vi "E816_Configuration_Setup No Password.vi"(0 "System no.":i32=1 min=1 step=1, 1 "Interface":u16(ring) items=["RS232", "USB"], 2 "Axes to move":string[](array[string]), 3 "All axes?":bool=TRUE, 4 "Change servo \nstatus to ON?":bool=TRUE, 5 "error in":errorcluster, 7 "Timeout":i32=5000, 8 "RS232 settings":cluster{"Portnumber":i32, "Baudrate":u16}={"Portnumber"=0, "Baudrate"=4} {"Portnumber" items=["COM1", "COM2", "COM3", "COM4", "COM5", "COM6", "COM7", "COM8", "COM9", "COM10", "COM11", "COM12", "COM13", "COM14", "COM15", "COM16", "COM17", "COM18", "COM19", "COM20", "COM21", "COM22", "COM23", "COM24", "COM25", "COM26", "COM27", "COM28", "COM29", "COM30"]; "Baudrate" items=["9600", "14400", "19200", "38400", "57600", "115200"]}, 9 "USB settings":cluster{"S/N":string, "USB Search?":bool}={"S/N"="", "USB Search?"=TRUE}, 13 "Stop refnum":refnum<vi>) -> (14 "Identification":string, 15 "SN out":string, 16 "Conn. Axes":string[](array[string]), 17 "Position":dbl[](array[numeric]) format="%.6f", 19 "error out":errorcluster)   [LabVIEW 2020]
doc: "This VI performs a fully automatic initialization of the selected system (global settings and servo status) in the LabVIEW environment. Use the Help?Show Context Help menu sequence in the LabVIEW environment to display the Context Help window with the VI and control/indicator descriptions.\n\nAfter the successful running of this VI, all command VIs are ready to use. Specify the correct parameters first: \n¢ System No.: 1 in a one-system-only configuration\n¢ Timeout value (in milliseconds)\n¢ Interface (RS232 or USB)\n¢ For Interface = RS232: RS-232 settings: Choose the port number the E-816 is connected to and an appropriate baud rate. \n¢ For Interface = USB: appropriate Serial Number of the controller to connect to or if you want to search for the controller.\n¢ Whether the servo status of all axes is to change to TRUE. If FALSE is selected here, the servo status will not be changed.\n\nThen start the VI.\n\"E816_Configuration_Setup.vi\" performs the following initialization tasks:\n1. Initializes all global variables.\n2. Runs \"PI Open Interface of one system.vi\" to open a connection to the controller. \n3. Runs \"*IDN?.vi\" to query for the controller identification string. \n4. Defines the selected system to be \"E-816\"\n5. Runs \"Define connected axes.vi\" with Read from controller = TRUE and Invert Order? = FALSE. \n6. Runs \"SVO.vi\" to switch servo ON for all connected axes if Change servo status to ON is TRUE.\n7. Runs \"SVO?.vi\" to query for the servo status of all connected axes.\n8. Runs \"POS?.vi\" to query for the position of all axes.\n9. Runs \"ERR?.vi\" to query the master controller for its error status.\n10. Runs \"GCSTranslateError.vi\" to append the error message which corresponds with a GCS error number returned by \"ERR?.vi\" to Source from Error out.\n\nUse this VI as the initialization VI for the E-816 in your application.\nWhen using as a sub-VI, connect Stop refnum terminal to stop VI from caller.\n\nAs the initialization is a complex procedure which uses a large number of sub-VIs, E816_Configuration_Setup.vi is password-protected, meaning that you cannot see or modify the diagram. In this way, the full initialization is packed into one single and fully tested procedure which you simply insert into your own application program. For security reasons as well as your convenience, we recommend that you not modify this VI."
uses:
  Low Level/Communication.llb/Available DLLs.ctl
  Low Level/Communication.llb/Available interfaces.ctl
  Low Level/Communication.llb/Available DLL interfaces.ctl
  Low Level/General command.llb/Controller names.ctl
  Low Level/Communication.llb/Global1.vi
panel:
  out "Servo status?":bool[](array[boolean])
  in  "Tab Control":enum32{"Interface settings", "Move settings"}(tab)
  in  "Frame":T1(ring)=enum."Open interface"
  in  "Finished":bool
  in  "stop":bool
  # "E-816 configuration setup program V6.0.2"
  # "This VI performs a full automatic initialization (global settings and servo status) for the\nselected system in the LabVIEW environment. After the successful run of this VI all \ncommand VIs are ready to use. Selectthe following settings first: interface settings and Move settings. See control/\nindicator information for details. Then start the VI. When using as a sub-VI, connect Stop refnum terminal to stop VI \nfrom caller.  See also VI information for details."
  # "Are all axes\nconnected\nand can be \nmoved?"
  # "If not:"
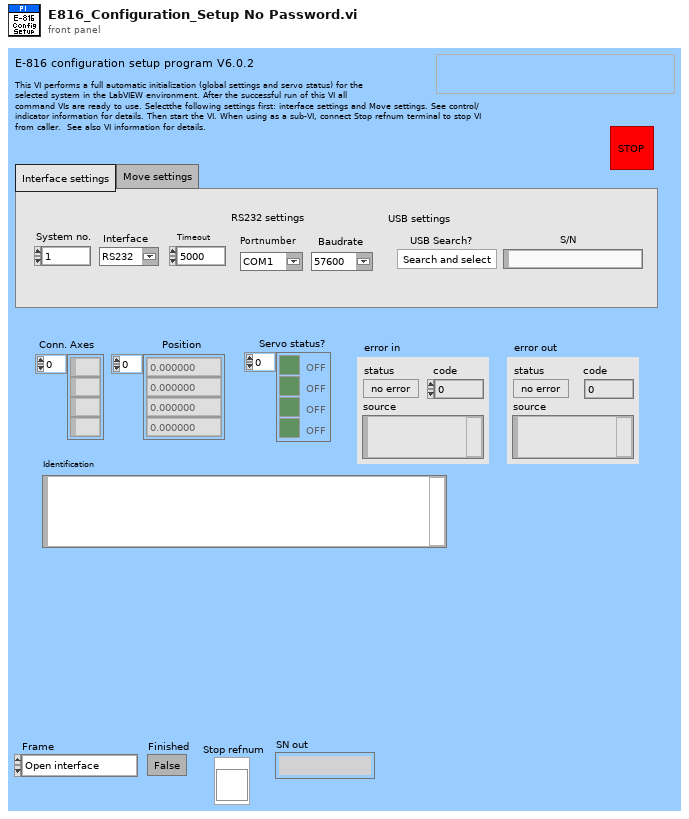
[diagram p1: front panel]
types:
  T1 = enum16{"Do nothing", "Initialize indicators", "Open interface", "Read IDs", "Set RON", "Reference", "Goto limit switch", "Move to middle", "Define home", "Translate error"}
  T2 = enum16{"DCO", "DCO?", "MOV", "MOV?", "MVR", "ONT?", "OVF?", "POS?", "RST", "SVA", "SVA?", "SVO", "SVO?", "SVR", "VOL?"}
  T3 = typedef "Available DLLs.ctl" = u16
  T4 = cluster{"input XON/XOFF":bool, "input HW Handshake":bool, "input alt HW HShk":bool, "output XON/XOFF":bool, "output HW Handshake":bool, "output alt HW HShk":bool, "XOFF byte ":u8, "XON byte":u8, "parity error byte":u16}[]
  T5 = typedef "Available DLL interfaces.ctl" = u16
  T6 = cluster{"input XON/XOFF":bool, "input HW Handshake":bool, "input alt HW HShk":bool, "output XON/XOFF":bool, "output HW Handshake":bool, "output alt HW HShk":bool, "XOFF byte ":u8, "XON byte":u8, "parity error byte":u16}
  T7 = typedef "Available interfaces.ctl" = u16
  T8 = cluster{"DLL for Device":T3, "DLL Interface":T5, "Parameter":string}[]
  T9 = cluster{"RS232 Portnumber":i32, "Timeout":i32, "RS232 Baud rate":u32, "Interface":T7, "GPIB Bus":i32, "GPIB Address":i32, "GPIB Mode":i32}[]
  T10 = cluster{"DLL for Device":T3, "DLL Interface":T5, "Parameter":string}
  T11 = cluster{"RS232 Portnumber":i32, "Timeout":i32, "RS232 Baud rate":u32, "Interface":T7, "GPIB Bus":i32, "GPIB Address":i32, "GPIB Mode":i32}
  T12 = typedef "Controller names.ctl" = enum16{"None", "Analog", "C-702", "C-843", "C-843.PM", "C-844", "C-848", "C-865", "C-866", "C-867", "C-880", "E-516", "E-517", "E-709", "E-710", "E-712", "E-725", "E-753", "E-755", "E-761", "E-816", "E-861", "F-206", "M-840", "M-850", "M-8X0", "Mercury", "Mercury_GCS"}
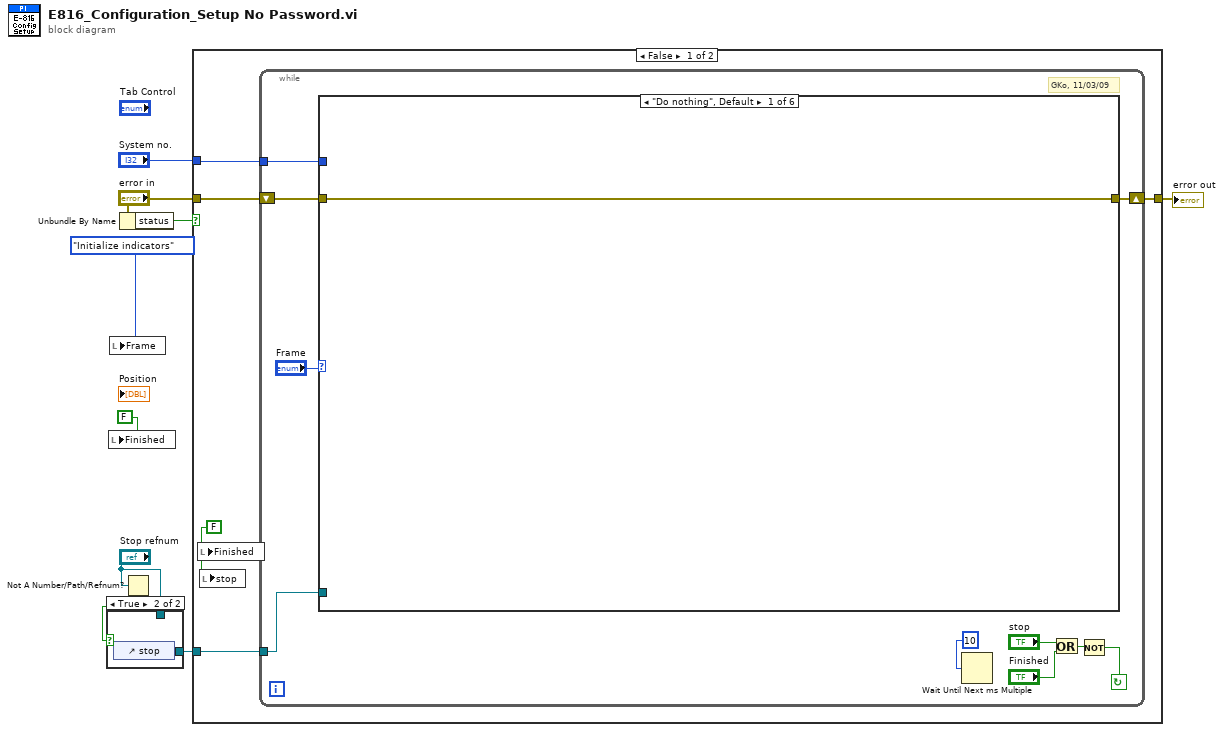
[diagram p0: block diagram]
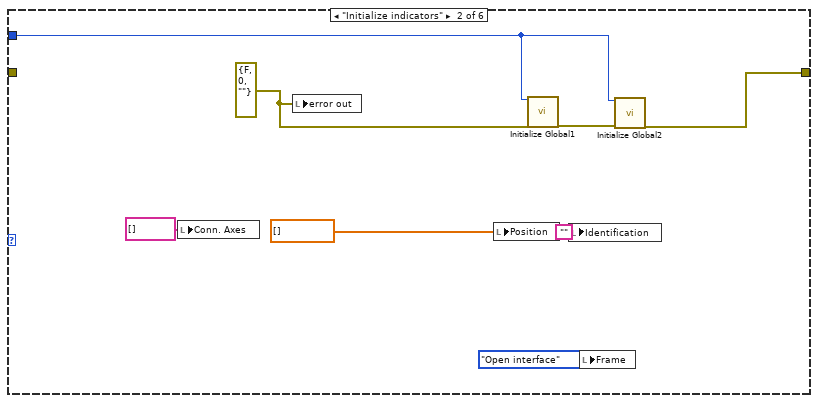
[diagram p3: hidden frame]
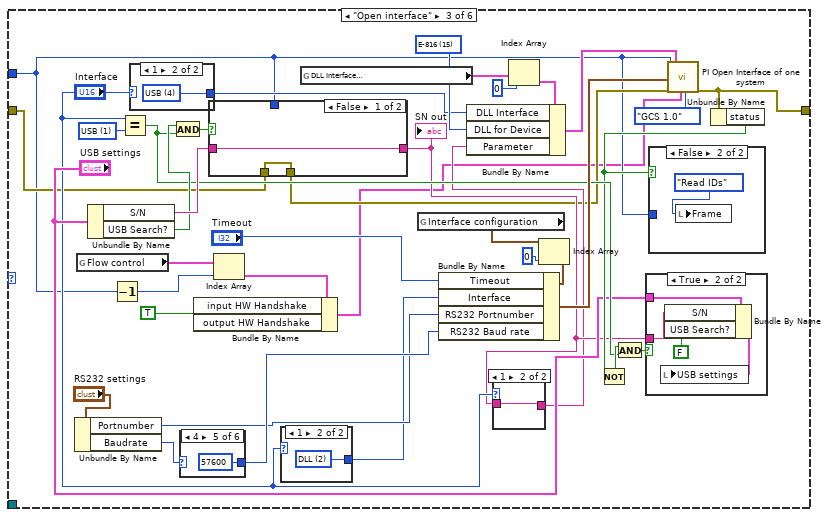
[diagram p4: hidden frame]
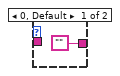
[diagram p5: hidden frame]
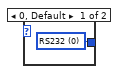
[diagram p6: hidden frame]
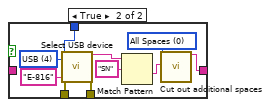
[diagram p8: hidden frame]
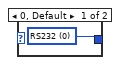
[diagram p9: hidden frame]
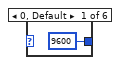
[diagram p10: hidden frame]
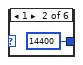
[diagram p11: hidden frame]
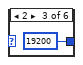
[diagram p12: hidden frame]
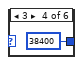
[diagram p13: hidden frame]
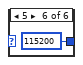
[diagram p14: hidden frame]
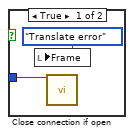
[diagram p15: hidden frame]
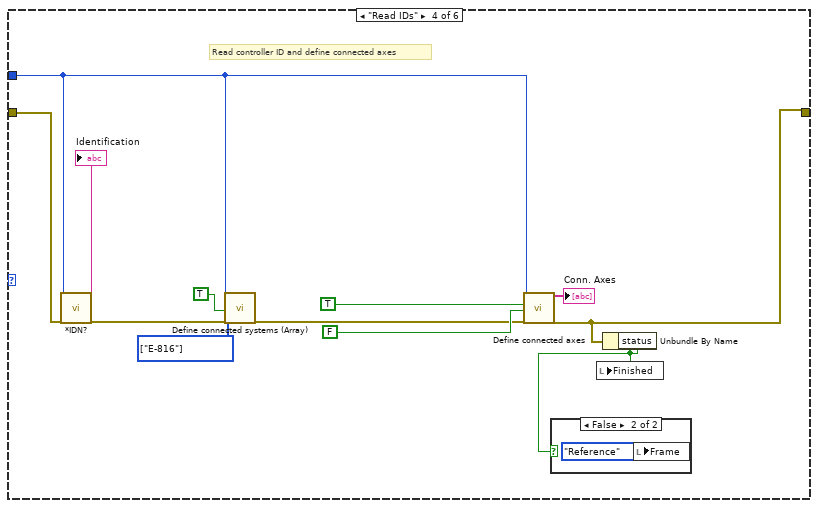
[diagram p16: hidden frame]
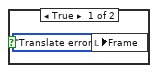
[diagram p17: hidden frame]
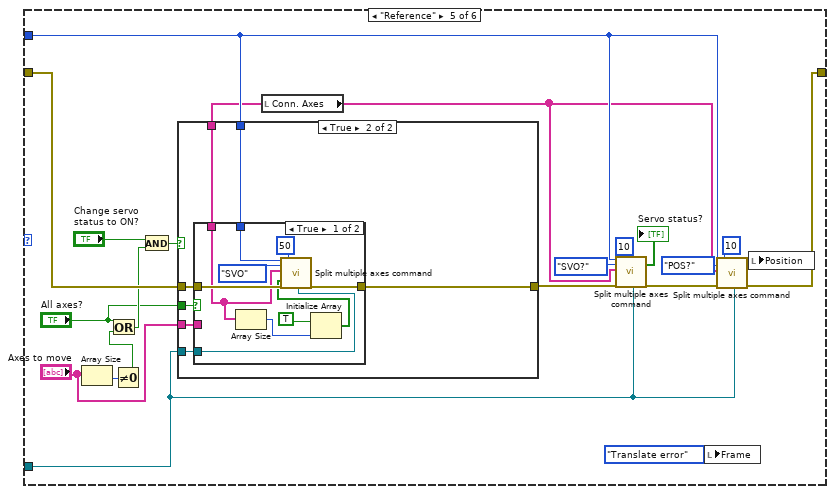
[diagram p18: hidden frame]
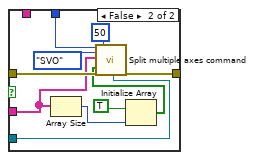
[diagram p20: hidden frame]
diagram:
  n1 = local write "Finished"(FALSE ("Finished")) -> ()
  n2 = local write "Frame"(T1."Initialize indicators" ("Frame")) -> ()
  n3 = Unbundle By Name("error in") -> ("status"=w8:bool)
  n4 = Not A Number/Path/Refnum?(number/path/refnum="Stop refnum") -> (NaN/Path/Refnum?=w4:bool)
  n5 = case shown="True" w4 {
    tunnel: [w10 w11] -> w2
    tunnel: "Stop refnum" -> [w10 _]
    frame False {
    }
    frame True {
      n6 = control-ref of="stop"() -> (w11:refnum<vi>)
    }
  }
  n7 = case shown="False" w8 {
    tunnel: [w15 w174] -> w6
    tunnel: "error in" -> [w16 w174]
    tunnel: "System no." -> [w14 _]
    tunnel: w2 -> [w12 _]
    frame False {
      w13 = FALSE ("Finished")
      n8 = local write "Finished"(w13) -> ()
      n9 = local write "stop"(w13) -> ()
      n10 = while {
        tunnel: w12 -> [w17]
        shift-left: w16 -> [w20]
        shift-right: [w19] -> w15
        tunnel: w14 -> [w18]
        stop <- w22 continue-if-true
        # "GKo, 11/03/09"
        n11 = case shown="\"Do nothing\", Default" "Frame" {
          tunnel: w18 -> [_ w29 w38 w107 w131 w169]
          tunnel: w20 -> [w27 _ w44 w110 w138 w172]
          tunnel: [w27 w30 w47 w106 w136 w170] -> w19
          tunnel: w17 -> [_ _ _ _ w124 _]
          frame "Do nothing", Default {
          }
          frame "Initialize indicators" {
            w31 = errorcluster {"status"=FALSE, "code"=0, "source"=""} ("error out")
            n12 = local write "Conn. Axes"(string[] [] ("Conn. Axes")) -> ()
            n13 = local write "error out"(w31) -> ()
            n14 = local write "Position"(dbl[] [] ("Position")) -> ()
            n15 = call "Initialize Global1.vi"("System no."=w29, "error in"=w31) -> ("error out"=w28:errorcluster)  [unwired: 17 in]
            n16 = local write "Identification"("" ("Identification")) -> ()
            n17 = local write "Frame"(T1."Open interface" ("Frame")) -> ()
            n18 = call "Initialize Global2.vi"("System no."=w29, "error in"=w28) -> ("error out"=w30:errorcluster)  [unwired: 17 in]
          }
          frame "Open interface" {
            w36 = u16 1 items=["RS232", "USB"] ("Interface")
            w64 = T3 15 items=["C-843", "C-844", "E-710", "C-843.PM", "C-865", "E-761", "Mercury", "E-755", "E-753", "C-866", "E-712", "E-725", "E-861", "C-867", "E-517", "E-816", "E-709", "PI_GCS2_DLL"] ("DLL for Device")
            w41 = TRUE ("Bundle Element")
            n19 = Unbundle By Name("RS232 settings") -> ("Portnumber"=w54:i32, "Baudrate"=w65:u16)
            n20 = global read "Global1.vi" "Flow control"() -> (w40:T4)
            n21 = Unbundle By Name("USB settings") -> ("S/N"=w63:string, "USB Search?"=w61:bool)
            n22 = Decrement(x=w38) -> (x-1=w39:i32)
            n23 = Equal?(x="Interface", y=w36) -> (x = y?=w57:bool)
            n24 = case shown="1" "Interface" {
              tunnel: [w94 w95] -> w56
              frame 0, Default {
                w94 = T5 0 items=["RS232", "GPIB", "Board", "TCP-IP", "USB", "RS232_DC"] ("DLL Interface")
              }
              frame 1 {
                w95 = T5 4 items=["RS232", "GPIB", "Board", "TCP-IP", "USB", "RS232_DC"] ("DLL Interface")
              }
            }
            n25 = And(x=w61, y=w57) -> (x .and. y?=w60:bool)
            n26 = case shown="4" w65 {
              tunnel: [9600 14400 19200 38400 57600 115200] -> w55
              frame 0, Default {
              }
              frame 1 {
              }
              frame 2 {
              }
              frame 3 {
              }
              frame 4 {
              }
              frame 5 {
              }
            }
            n27 = case shown="False" w60 {
              tunnel: [w83 w86] -> w49
              tunnel: w63 -> [w83 _]
              tunnel: w38 -> [_ w93]
              tunnel: w44 -> [w82 w90]
              tunnel: [w82 w89] -> w43
              frame False {
              }
              frame True {
                w87 = u16 0 items=["All Spaces", "Only if 1st char.", "Only if last char.", "Only if near \"=\"", "Only if 1st or last char.", "Only multiple", "Really all"] ("Mode")
                w92 = T5 4 items=["RS232", "GPIB", "Board", "TCP-IP", "USB", "RS232_DC"] ("DLL Interface")
                n28 = call "Select USB device.vi"("System no."=w93, "DLL Interface"=w92, "Controller name"="E-816", "error in"=w90) -> ("Selected USB controller"=w85:string, "error out"=w89:errorcluster)  [unwired: 13 in, 1 out]
                n29 = Match Pattern(string=w85, regular expression="SN") -> (after substring=w88:string)  [unwired: 4 out]
                n30 = call "Cut out additional spaces.vi"("String"=w88, "Mode"=w87) -> ("String out"=w86:string)  [unwired: 17 out]
              }
            }
            "SN out" <- w49
            n31 = Index Array(array=w40, index=w39) -> (element=w42:T6)
            n32 = Bundle By Name(cluster=w42, "input HW Handshake"=w41, "output HW Handshake"=w41) -> (w37:T6)
            n33 = case shown="1" "Interface" {
              tunnel: [w76 w77] -> w52
              frame 0, Default {
                w76 = T7 0 items=["RS232", "GPIB", "DLL", "TCP-IP", "USB", "Analog"] ("Interface")
              }
              frame 1 {
                w77 = T7 2 items=["RS232", "GPIB", "DLL", "TCP-IP", "USB", "Analog"] ("Interface")
              }
            }
            n34 = global read "Global1.vi" "DLL Interface\nConfiguration"() -> (w71:T8)
            n35 = global read "Global1.vi" "Interface configuration"() -> (w68:T9)
            n36 = case shown="1" "Interface" {
              tunnel: w49 -> [_ w75]
              tunnel: ["" w75] -> w48
              frame 0, Default {
              }
              frame 1 {
              }
            }
            n37 = Index Array(array=w71, index=0 ("Index")) -> (element=w72:T10)
            n38 = Bundle By Name(cluster=w72, "DLL Interface"=w56, "DLL for Device"=w64, "Parameter"=w48) -> (w67:T10)
            n39 = Index Array(array=w68, index=0 ("Index")) -> (element=w73:T11)
            n40 = Bundle By Name(cluster=w73, "Timeout"="Timeout", "Interface"=w52, "RS232 Portnumber"=w54, "RS232 Baud rate"=w55) -> (w66:T11)
            n41 = call "PI Open Interface of one system.vi"("System number"=w38, "Interface configuration"=w66, "error in"=w43, "DLL Interface\nConfiguration"=w67, "Flow control"=w37, "Syntax"=enum16{"GCS 1.0", "GCS 2.0"}."GCS 1.0") -> ("error out"=w47:errorcluster)  [unwired: 6 in, 7 out]
            n42 = Unbundle By Name(w47) -> ("status"=w53:bool)
            n43 = Not(x=w53) -> (.not. x?=w59:bool)
            n44 = And(x=w59, y=w57) -> (x .and. y?=w58:bool)
            n45 = case shown="True" w58 {
              tunnel: "USB settings" -> [_ w81]
              tunnel: w49 -> [_ w79]
              frame False {
              }
              frame True {
                n46 = Bundle By Name(cluster=w81, "S/N"=w79, "USB Search?"=FALSE) -> (w78:cluster{"S/N":string, "USB Search?":bool})
                n47 = local write "USB settings"(w78) -> ()
              }
            }
            n48 = case shown="False" w53 {
              tunnel: w38 -> [w103 _]
              frame True {
                n49 = local write "Frame"(T1."Translate error" ("Frame")) -> ()
                n50 = call "Close connection if open.vi"("System no."=w103) -> ()  [unwired: 17 in, 2 out]
              }
              frame False {
                n51 = local write "Frame"(T1."Read IDs" ("Frame")) -> ()
              }
            }
          }
          frame "Read IDs" {
            w105 = T12[] [enum."E-816"] items=["None", "Analog", "C-702", "C-843", "C-843.PM", "C-844", "C-848", "C-865", "C-866", "C-867", "C-880", "E-516", "E-517", "E-709", "E-710", "E-712", "E-725", "E-753", "E-755", "E-761", "E-816", "E-861", "F-206", "M-840", "M-850", "M-8X0", "Mercury", "Mercury_GCS"] ("Controller names")
            # "Read controller ID and define connected axes"
            n52 = call "*IDN?.vi"("System no."=w107, "error in"=w110) -> ("Identification"=→"Identification":string, "error out"=w112:errorcluster)  [unwired: 16 in]
            n53 = call "Define connected systems (Array).vi"("System no."=w107, "Controller names"=w105, "Change only one system?"=TRUE, "error in"=w112) -> ("error out"=w108:errorcluster)  [unwired: 15 in]
            n54 = call "Define connected axes.vi"("System no."=w107, "Read from\ncontroller?"=TRUE ("Read from\nController"), "Invert\norder?"=FALSE ("Invert\norder?"), "error in"=w108) -> ("Conn. Axes out"=→"Conn. Axes":string[], "error out"=w106:errorcluster)  [unwired: 14 in]
            n55 = Unbundle By Name(w106) -> ("status"=w111:bool)
            n56 = case shown="False" w111 {
              frame True {
                n57 = local write "Frame"(T1."Translate error" ("Frame")) -> ()
              }
              frame False {
                n58 = local write "Frame"(T1."Reference" ("Frame")) -> ()
              }
            }
            n59 = local write "Finished"(w111) -> ()
          }
          frame "Reference" {
            n60 = Array Size(array="Axes to move") -> (size(s)=w123:i32)
            n61 = Not Equal To 0?(x=w123) -> (x != 0?=w122:bool)
            n62 = Or(x="All axes?", y=w122) -> (x .or. y?=w121:bool)
            n63 = And(x="Change servo \nstatus to ON?", y=w121) -> (x .and. y?=w134:bool)
            n64 = local read "Conn. Axes"() -> (w130:string[])
            n65 = case shown="True" w134 {
              tunnel: [w140 w146] -> w132
              tunnel: w138 -> [w140 w147]
              tunnel: w130 -> [_ w144]
              tunnel: w131 -> [_ w145]
              tunnel: w124 -> [_ w143]
              tunnel: "All axes?" -> [_ w142]
              tunnel: "Axes to move" -> [_ w141]
              frame False {
              }
              frame True {
                n66 = case shown="True" w142 {
                  tunnel: w147 -> [w157 w167]
                  tunnel: [w156 w166] -> w146
                  tunnel: w145 -> [w155 w165]
                  tunnel: w144 -> [w153 _]
                  tunnel: w143 -> [w149 w160]
                  tunnel: w141 -> [_ w158]
                  frame True {
                    n67 = Array Size(array=w153) -> (size(s)=w152:i32)
                    n68 = Initialize Array(TRUE, w152) -> (w150:bool[])
                    n69 = call "Split multiple axes command.vi"("System no."=w155, "Command"=T2."SVO", "Axes to command"=w153, "Bool. values in"=w150, "error in"=w157, "Wait time (ms)"=u32 50 ("Wait time"), "Stop refnum"=w149) -> ("error out"=w156:errorcluster)  [unwired: 10 in, 2 out]
                  }
                  frame False {
                    n70 = Array Size(array=w158) -> (size(s)=w163:i32)
                    n71 = Initialize Array(TRUE, w163) -> (w161:bool[])
                    n72 = call "Split multiple axes command.vi"("System no."=w165, "Command"=T2."SVO", "Axes to command"=w158, "Bool. values in"=w161, "error in"=w167, "Wait time (ms)"=u32 50 ("Wait time"), "Stop refnum"=w160) -> ("error out"=w166:errorcluster)  [unwired: 2 in, 10 out]
                  }
                }
              }
            }
            n73 = call "Split multiple axes command.vi"("System no."=w131, "Command"=T2."SVO?", "Axes to command"=w130, "error in"=w132, "Wait time (ms)"=u32 10 ("Wait time"), "Stop refnum"=w124) -> ("Bool. values out"=→"Servo status?":bool[], "error out"=w128:errorcluster)  [unwired: 3 in, 9 out]
            n74 = local write "Frame"(T1."Translate error" ("Frame")) -> ()
            n75 = call "Split multiple axes command.vi"("System no."=w131, "Command"=T2."POS?", "Axes to command"=w130, "error in"=w128, "Wait time (ms)"=u32 10 ("Wait time"), "Stop refnum"=w124) -> ("Num. values out"=w139:dbl[], "error out"=w136:errorcluster)  [unwired: 3 in, 9 out]
            n76 = local write "Position"(w139) -> ()
          }
          frame "Translate error" {
            n77 = call "ERR?.vi"("System no."=w169, "error in"=w172) -> ("error out"=w171:errorcluster)  [unwired: 16 in, 1 out]
            n78 = local write "Finished"(TRUE ("Finished")) -> ()
            n79 = call "GCSTranslateError.vi"("error in"=w171) -> ("error out"=w170:errorcluster)  [unwired: 18 out]
            n80 = local write "Frame"(T1."Do nothing" ("Frame")) -> ()
          }
        }
        n81 = Wait Until Next ms Multiple(millisecond multiple=u32 10) -> ()  [unwired: 1 out]
        n82 = Or(x="stop", y="Finished") -> (x .or. y?=w24:bool)
        n83 = Not(x=w24) -> (.not. x?=w22:bool)
      }
    }
    frame True {
    }
  }
  "error out" <- w6
